vi "Memory.Pointer.Set Address.vi"(8 "error in (no error)":errorcluster, 10 "address":u64 format="%016x", 11 "Pointer in":refnum<class "Memory.Pointer.Void.lvclass">) -> (0 "error out":errorcluster, 3 "Pointer out":refnum<class "Memory.Pointer.Void.lvclass">)   [LabVIEW 2016, in "Memory Manager.lvlib" / "Memory.Pointer.Void.lvclass"]
uses:
  Memory.Pointer.Void.lvclass
  Memory.Pointer.Void.lvclass/Memory.Pointer.Void.ctl
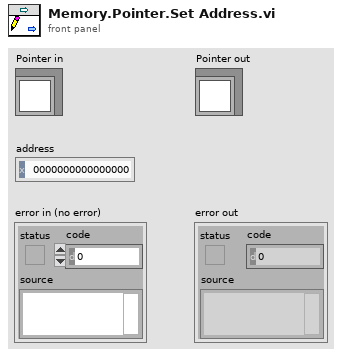
[diagram p1: front panel]
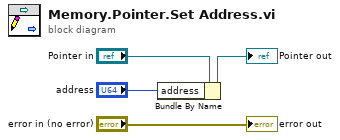
[diagram p0: block diagram]
diagram:
  n1 = Bundle By Name(cluster="Pointer in", "address"="address") -> (→"Pointer out":refnum<class "Memory.Pointer.Void.lvclass">)
  "error out" <- "error in (no error)"
